vi "Drive.vi"   [LabVIEW 2012]
uses:
  StateMachineEnum.ctl
  <vilib>/Rock Robotics/WPI/RobotDrive/WPI_RobotDriveGetSetRefNum.vi
  Robot Global Data.vi
types:
  T1 = typedef "StateMachineEnum.ctl" = enum16{"Init", "Idle", "Start", "Do", "Stop"}
  T2 = typedef "WPI_RobotDriveDevRef.ctl" = cluster{"DevStatus":errorcluster, "Motors[]":T3[], "Square Inputs":bool, "Max Output":dbl, "Isochronous":bool}
  T3 = typedef "WPI_MotorControlDeviceRef.ctl" = cluster{"DeviceStatus":errorcluster, "Type":enum16{"PWM", "CAN"}, "PWM":cluster{"Digital Module":T4, "PWM Channel":T5, "DeadBand":T6}, "CAN":cluster{"Device Number":u8, "Control Mode":T7, "Semaphore":T8, "Max Vout":dbl}, "Invert":bool, "TransformRef":T9, "InvTransformRef":T9}
  T4 = typedef "FPGA_TypedefDigitalModule.ctl" = enum16{"Digital Module 1", "Digital Module 2"}
  T5 = typedef "FPGA_DIOPWMChannel.ctl" = enum8{"PWM 1", "PWM 2", "PWM 3", "PWM 4", "PWM 5", "PWM 6", "PWM 7", "PWM 8", "PWM 9", "PWM 10", "Invalid"}
  T6 = typedef "WPI_PWMDeadband.ctl" = cluster{"Name":string, "maxPositivePwm":i32, "minPositivePwm":i32, "centerPwm":i32, "maxNegativePwm":i32, "minNegativePwm":i32, "angularRange":u16}
  T7 = typedef "WPI_CANJaguar_ControlMode.ctl" = enum8{"Percent VBus", "Current", "Speed", "Position", "Voltage"}
  T8 = typedef "Semaphore RefNum" = refnum<k1>
  T9 = typedef "WPI_PWMTransform_ConPane.ctl" = refnum<vi>
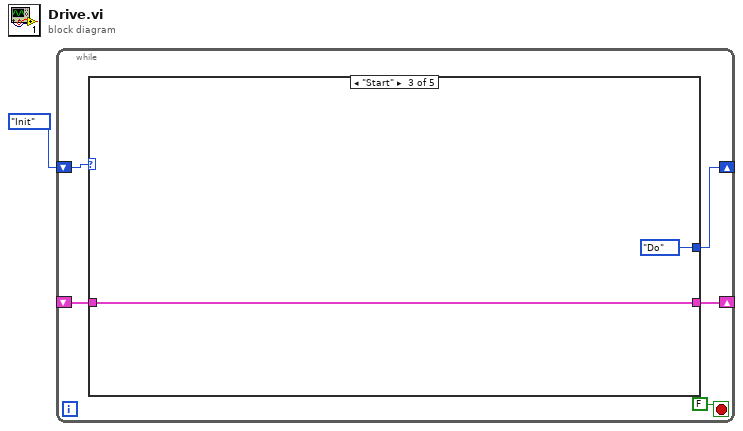
[diagram p0: block diagram]
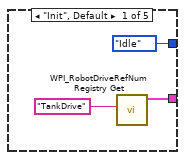
[diagram p2: hidden frame]
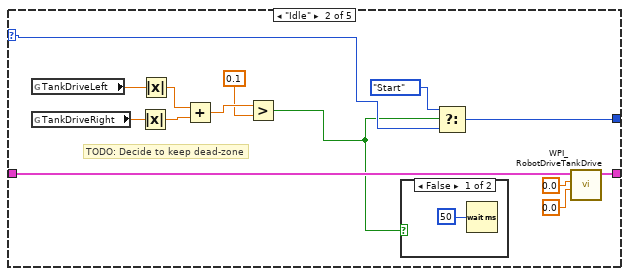
[diagram p3: hidden frame]
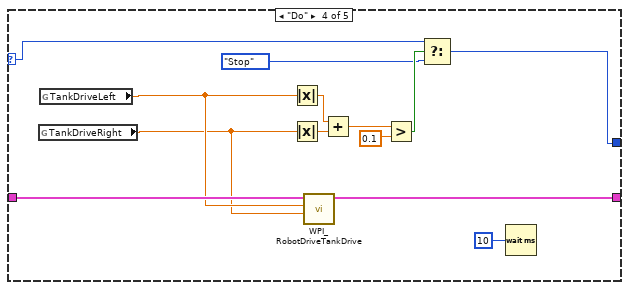
[diagram p5: hidden frame]
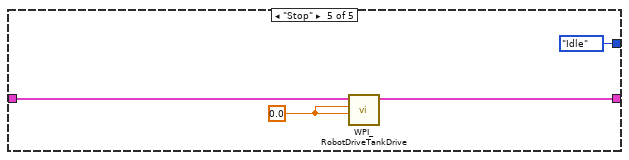
[diagram p6: hidden frame]
diagram:
  n1 = while {
    shift-right: [w2] -> _
    shift-left: StateMachineEnum."Init" -> [w5]
    shift-right: [w4] -> _
    shift-left: _ -> [w3]
    stop <- FALSE stop-if-true
    n2 = case shown="\"Start\"" w5 {
      selector: w5 -> [_ w11 _ w34 _]
      tunnel: [w8 w12 w25 w30 w42] -> w4
      tunnel: w3 -> [_ w14 w25 w31 w43]
      tunnel: [StateMachineEnum."Idle" w19 StateMachineEnum."Do" w32 StateMachineEnum."Idle" ("f")] -> w2
      frame "Init", Default {
        n3 = call <vilib>:"WPI_RobotDriveRefNum Registry Get.vi"("refnum name"="TankDrive") -> ("RobotDriveDevRef"=w8:T2)  [unwired: 9 in, 1 out]
      }
      frame "Idle" {
        # "TODO: Decide to keep dead-zone"
        n4 = global read "Robot Global Data.vi" "TankDriveLeft"() -> (w15:dbl)
        n5 = global read "Robot Global Data.vi" "TankDriveRight"() -> (w16:dbl)
        n6 = Absolute Value(x=w16) -> (abs(x)=w22:dbl)
        n7 = Absolute Value(x=w15) -> (abs(x)=w23:dbl)
        n8 = Add(x=w23, y=w22) -> (x+y=w21:dbl)
        n9 = Greater?(x=w21, y=0.1) -> (0:w10:bool)
        n10 = case shown="False" w10 {
          frame False {
            n11 = Wait (ms)(milliseconds to wait=u32 50) -> ()  [unwired: 1 out]
          }
          frame True {
          }
        }
        n12 = Select(t=StateMachineEnum."Start", s=w10, f=w11) -> (s? t:f=w19:T1)
        n13 = call <vilib>:"WPI_RobotDriveTankDrive.vi"("Right axis value"=0.0, "Left axis value"=0.0, "RobotDriveDevRef"=w14) -> ("RobotDriveDevRef"=w12:T2)  [unwired: 6 in, 2 out]
      }
      frame "Start" {
      }
      frame "Do" {
        n14 = global read "Robot Global Data.vi" "TankDriveRight"() -> (w28:dbl)
        n15 = global read "Robot Global Data.vi" "TankDriveLeft"() -> (w29:dbl)
        n16 = Absolute Value(x=w29) -> (abs(x)=w39:dbl)
        n17 = Absolute Value(x=w28) -> (abs(x)=w38:dbl)
        n18 = call <vilib>:"WPI_RobotDriveTankDrive.vi"("Right axis value"=w28, "Left axis value"=w29, "RobotDriveDevRef"=w31) -> ("RobotDriveDevRef"=w30:T2)  [unwired: 6 in, 2 out]
        n19 = Add(x=w39, y=w38) -> (x+y=w36:dbl)
        n20 = Greater?(x=w36, y=0.1) -> (0:w35:bool)
        n21 = Select(t=w34, s=w35, f=StateMachineEnum."Stop") -> (s? t:f=w32:T1)
        n22 = Wait (ms)(milliseconds to wait=u32 10) -> ()  [unwired: 1 out]
      }
      frame "Stop" {
        w41 = 0.0 ("Left axis value")
        n23 = call <vilib>:"WPI_RobotDriveTankDrive.vi"("Right axis value"=w41, "Left axis value"=w41, "RobotDriveDevRef"=w43) -> ("RobotDriveDevRef"=w42:T2)  [unwired: 6 in, 2 out]
      }
    }
  }
